vi "add_message.vi"(8 "error in (no error)":errorcluster, 10 "message string":string, 11 "Message in":refnum<class "Message.lvclass">) -> (0 "error out":errorcluster, 3 "Message out":refnum<class "Message.lvclass">)   [LabVIEW 2017, in "Message.lvclass"]
doc: "adds a message to \"current message\", the time string is created automatially. It also adds the message to the \"message history\"."
uses:
  Message.lvclass
  Message.lvclass/Message.ctl
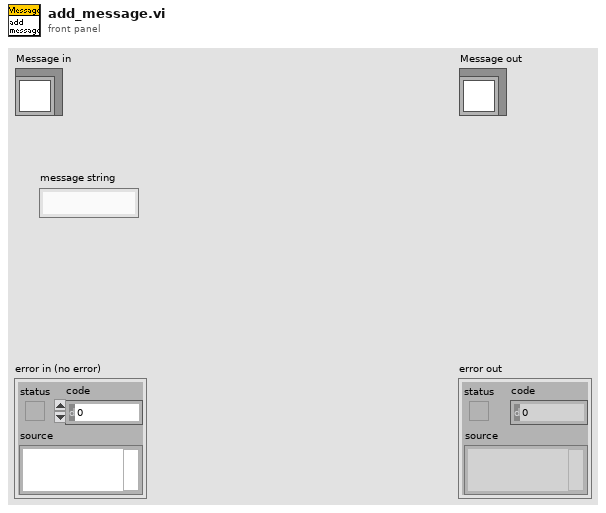
[diagram p1: front panel]
types:
  T1 = cluster{"time string":string, "message":string}[]
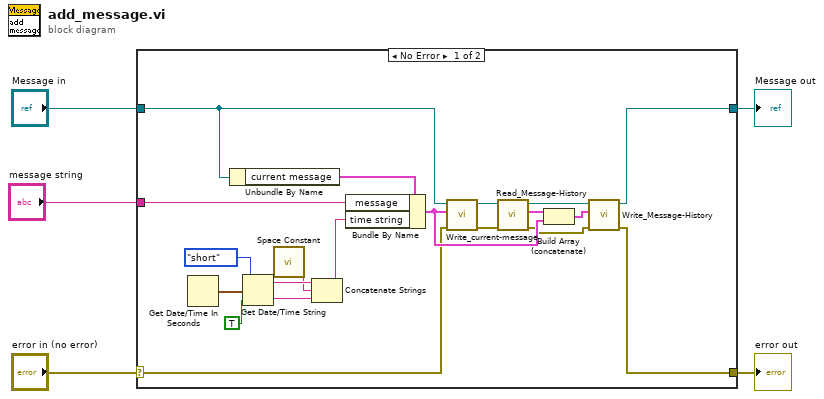
[diagram p0: block diagram]
diagram:
  n1 = case shown="No Error" "error in (no error)" {
    selector: "error in (no error)" -> [w7 w27]
    tunnel: [w6 w27] -> w4
    tunnel: [w8 w26] -> w2
    tunnel: "Message in" -> [w19 w26]
    tunnel: "message string" -> [w16 _]
    frame No Error {
      n2 = Get Date/Time In Seconds() -> (seconds since 1Jan1904=w25:timestamp)
      n3 = Unbundle By Name(w19) -> ("current message"=w18:cluster{"time string":string, "message":string})
      n4 = Get Date/Time String(date format (0)=enum16{"short", "long", "abbreviated"}."short", seconds (now)=w25, want seconds? (F)=TRUE) -> (date string=w22:string, time string=w20:string)
      n5 = call <vilib>:"Space Constant.vi"() -> ("String"=w21:string)
      n6 = Concatenate Strings(w22, w21, w20) -> (w17:string)
      n7 = Bundle By Name(cluster=w18, "message"=w16, "time string"=w17) -> (w12:cluster{"time string":string, "message":string})
      n8 = call "Write_current-message.vi"("error in (no error)"=w7, "current message"=w12, "Message in"=w19) -> ("error out"=w14:errorcluster, "Message out"=w15:refnum<class "Message.lvclass">)  [unwired: 7 in]
      n9 = call "Read_Message-History.vi"("error in (no error)"=w14, "Message in"=w15) -> ("error out"=w10:errorcluster, "message history"=w13:T1, "Message out"=w11:refnum<class "Message.lvclass">)  [unwired: 7 in]
      n10 = Build Array (concatenate)(w13, w12) -> (w9:T1)
      n11 = call "Write_Message-History.vi"("error in (no error)"=w10, "message history"=w9, "Message in"=w11) -> ("error out"=w6:errorcluster, "Message out"=w8:refnum<class "Message.lvclass">)  [unwired: 7 in]
    }
    frame Error {
    }
  }
  "error out" <- w4
  "Message out" <- w2
